vi "test String to Byte_2.vi"(11 "Test Case In":refnum<class "test EDS.lvclass">) -> (0 "error out":errorcluster, 3 "Test Case Out":refnum<class "test EDS.lvclass">)   [LabVIEW 2024, in "test EDS.lvclass"]
uses:
  test EDS.lvclass
  C:/Program Files/National Instruments/LabVIEW 2024/vi.lib/Astemes/LUnit/Test Case.lvclass
  <vilib>/Astemes/LUnit/Test Case.lvclass/Test Case.ctl
  <vilib>/Astemes/LUnit/Append Fail Result.vi
  <vilib>/Astemes/LUnit/Append Pass Result.vi
  <vilib>/Astemes/LUnit/Run In UI.vi
  <vilib>/Utility/error.llb/Clear Errors.vi
  Core/EDS.lvlib
  <vilib>/Astemes/LUnit/Test Case.lvclass
panel:
  out "Byte":u8
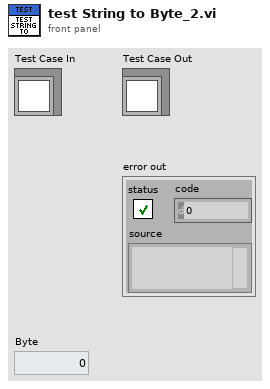
[diagram p1: front panel]
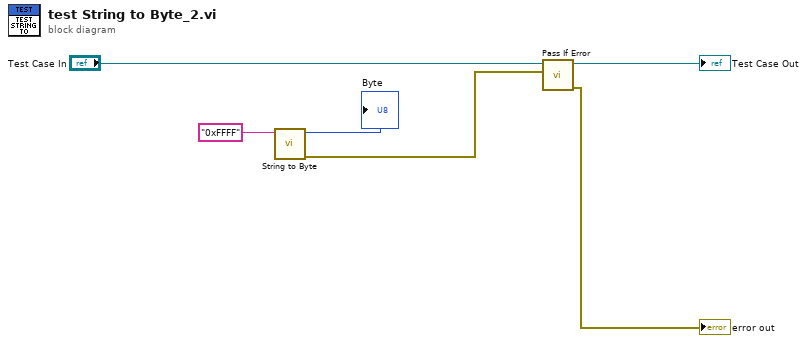
[diagram p0: block diagram]
diagram:
  n1 = call "String to Byte.vi"("String"="0xFFFF") -> ("error out"=w2:errorcluster, "Byte"=→"Byte":u8)  [unwired: 9 in]
  n2 = call <vilib>:"Pass If Error.vi"("Assert error"=w2, "LUnit Test Case In"="Test Case In") -> ("error out"=→"error out":errorcluster, "LUnit Test Case Out"=→"Test Case Out":refnum<class "test EDS.lvclass">)  [unwired: 8 in]
